vi "Find Gamma.vi"(8 "error in (no error)":errorcluster, 10 "IK Parameters":T2, 11 "Data in":T1={"link 1 angle"=0.0, "link 2 angle"=0.0, "link 1 length"=0.0, "link 2 length"=0.0, "Current arm location"=[{"X"=0.0, "Y"=0.0}, {"X"=-37.249783598972314, "Y"=33.353464914904016}, {"X"=-74.49956719794463, "Y"=66.70692982980803}], "Link Picture"=bytes[1162], "Desired Location"={"Desired X"=0.0, "Desired Y"=0.0}, "Next Location"={"Next X"=0.0, "Next Y"=0.0}, "Error"={"Joint1 error"=0.0, "Joint2 error"=0.0}, "tdms data"=refnum, "de/dt"={"joint1 de/dt"=0.0, "joint2 de/dt"=0.0}, "Voltages"={"Joint1 voltage"=0.0, "Joint2 voltage"=0.0}, "Time"=0.0, "dt"=0.0, "counts/rev"=0.0, "kp"=0.0, "kd"=0.0, "ki"=0.0, "Int(error)"={"joint1 int(e)"=0.0, "joint2 int(e)"=0.0}, "Desired angles"={"theta 1"=0.0, "theta 2"=0.0}, "Current counts"={"theta 1"=0.0, "theta 2"=0.0}, "Desired Counts"={"theta 1"=0.0, "theta 2"=0.0}, "Preivous Error"={"Joint1 Previous error"=0.0, "Joint2 Previous error"=0.0}, "Counts/s"=0.0, "Correct counter"=0}) -> (0 "error out":errorcluster, 2 "IK Parameters Out":T2, 3 "Data Out":T1={"link 1 angle"=0.0, "link 2 angle"=0.0, "link 1 length"=0.0, "link 2 length"=0.0, "Current arm location"=[{"X"=0.0, "Y"=0.0}, {"X"=-37.249783598972314, "Y"=33.353464914904016}, {"X"=-74.49956719794463, "Y"=66.70692982980803}], "Link Picture"=bytes[1162], "Desired Location"={"Desired X"=0.0, "Desired Y"=0.0}, "Next Location"={"Next X"=0.0, "Next Y"=0.0}, "Error"={"Joint1 error"=0.0, "Joint2 error"=0.0}, "tdms data"=refnum, "de/dt"={"joint1 de/dt"=0.0, "joint2 de/dt"=0.0}, "Voltages"={"Joint1 voltage"=0.0, "Joint2 voltage"=0.0}, "Time"=0.0, "dt"=0.0, "counts/rev"=0.0, "kp"=0.0, "kd"=0.0, "ki"=0.0, "Int(error)"={"joint1 int(e)"=0.0, "joint2 int(e)"=0.0}, "Desired angles"={"theta 1"=0.0, "theta 2"=0.0}, "Current counts"={"theta 1"=0.0, "theta 2"=0.0}, "Desired Counts"={"theta 1"=0.0, "theta 2"=0.0}, "Preivous Error"={"Joint1 Previous error"=0.0, "Joint2 Previous error"=0.0}, "Counts/s"=0.0, "Correct counter"=0})   [LabVIEW 2016]
uses:
  Type Defs/IK parameters.ctl
  Type Defs/Host Data.ctl
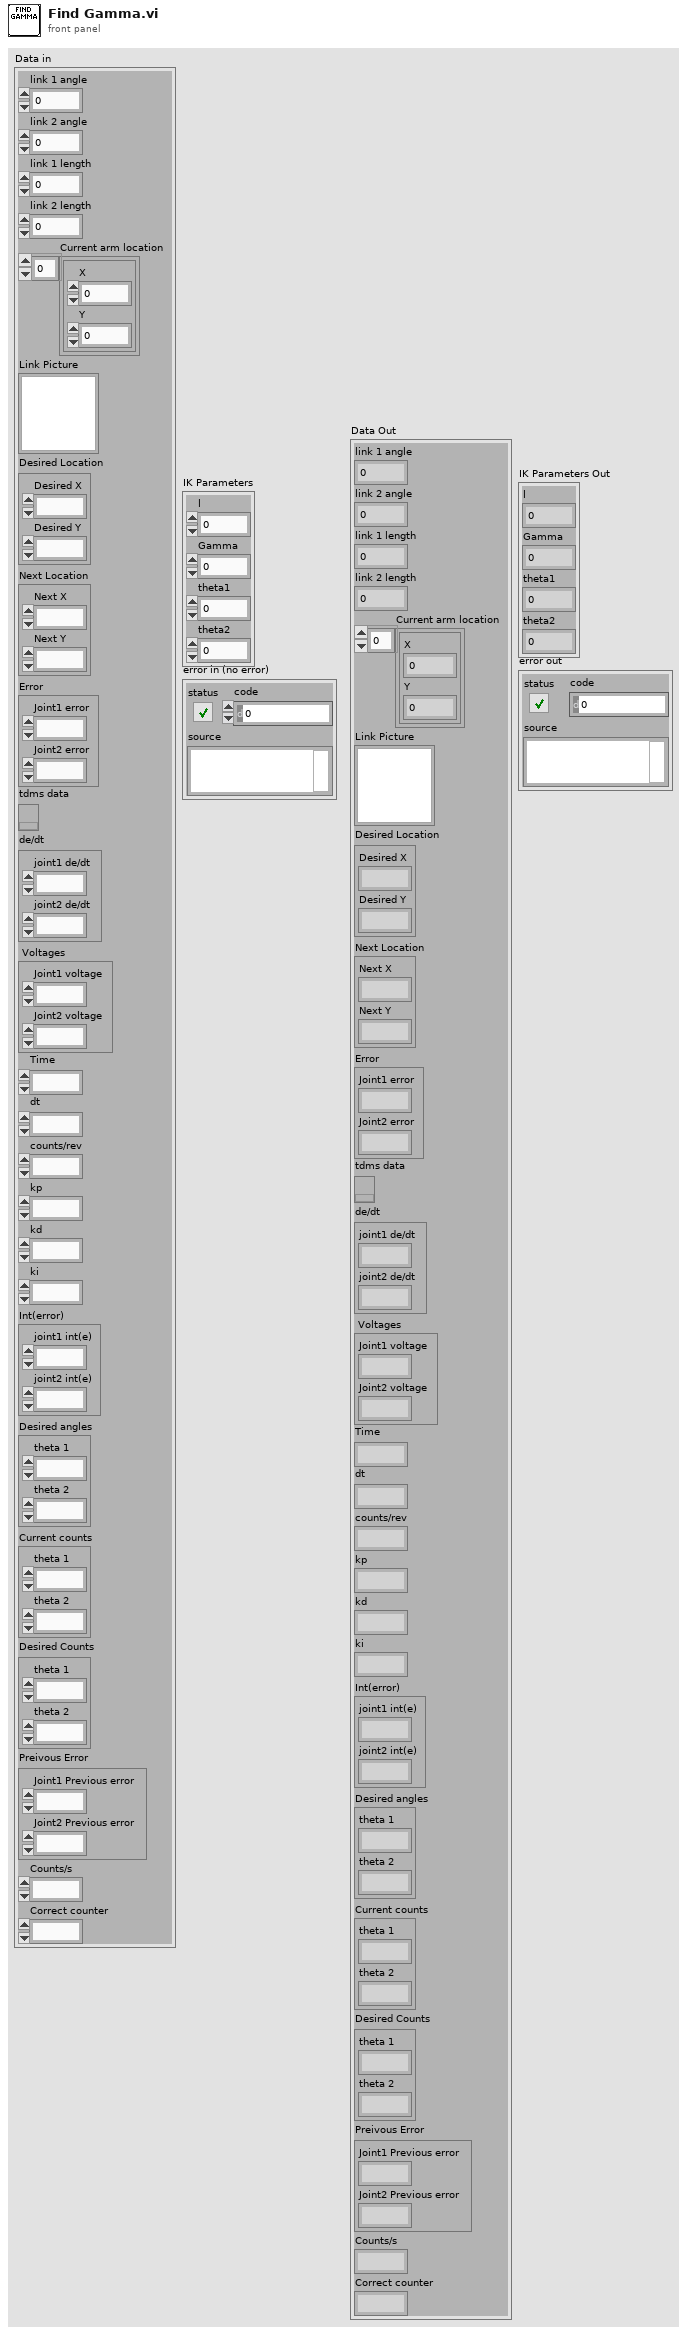
[diagram p1: front panel]
types:
  T1 = typedef "Host Data.ctl" = cluster{"link 1 angle":dbl, "link 2 angle":dbl, "link 1 length":dbl, "link 2 length":dbl, "Current arm location":cluster{"X":dbl, "Y":dbl}[], "Link Picture":picture, "Desired Location":cluster{"Desired X":dbl, "Desired Y":dbl}, "Next Location":cluster{"Next X":dbl, "Next Y":dbl}, "Error":cluster{"Joint1 error":dbl, "Joint2 error":dbl}, "tdms data":refnum<k34>, "de/dt":cluster{"joint1 de/dt":dbl, "joint2 de/dt":dbl}, "Voltages":cluster{"Joint1 voltage":dbl, "Joint2 voltage":dbl}, "Time":dbl, "dt":dbl, "counts/rev":dbl, "kp":dbl, "kd":dbl, "ki":dbl, "Int(error)":cluster{"joint1 int(e)":dbl, "joint2 int(e)":dbl}, "Desired angles":cluster{"theta 1":dbl, "theta 2":dbl}, "Current counts":cluster{"theta 1":dbl, "theta 2":dbl}, "Desired Counts":cluster{"theta 1":dbl, "theta 2":dbl}, "Preivous Error":cluster{"Joint1 Previous error":dbl, "Joint2 Previous error":dbl}, "Counts/s":dbl, "Correct counter":i32}
  T2 = typedef "IK parameters.ctl" = cluster{"l":dbl, "Gamma":dbl, "theta1":dbl, "theta2":dbl}
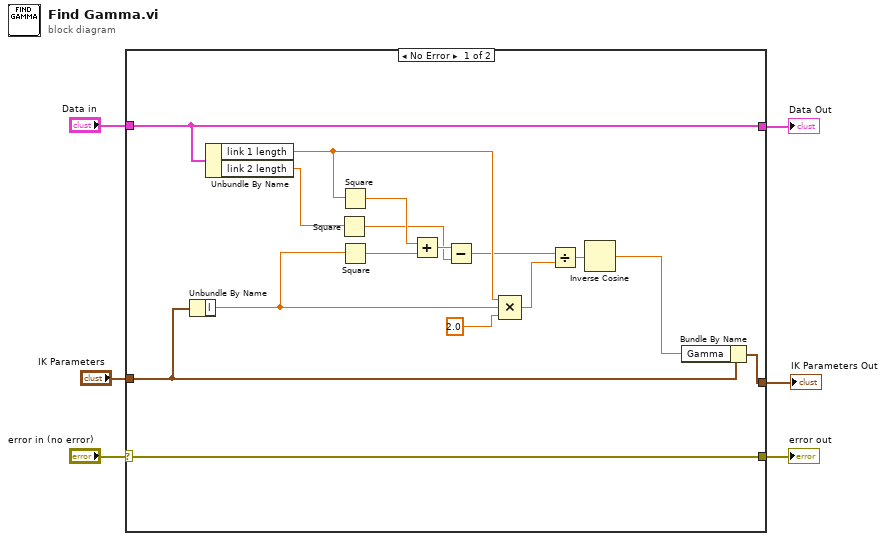
[diagram p0: block diagram]
diagram:
  n1 = case shown="No Error" "error in (no error)" {
    selector: "error in (no error)" -> [w21 w25]
    tunnel: [w21 w25] -> w5
    tunnel: "Data in" -> [w22 w24]
    tunnel: "IK Parameters" -> [w8 w23]
    tunnel: [w22 w24] -> w2
    tunnel: [w7 w23] -> w1
    frame No Error {
      n2 = Unbundle By Name(w8) -> ("l"=w14:dbl)
      n3 = Unbundle By Name(w22) -> ("link 1 length"=w15:dbl, "link 2 length"=w20:dbl)
      n4 = Square(x=w20) -> (x^2=w16:dbl)
      n5 = Square(x=w15) -> (x^2=w19:dbl)
      n6 = Square(x=w14) -> (x^2=w18:dbl)
      n7 = Add(x=w19, y=w18) -> (x+y=w17:dbl)
      n8 = Subtract(x=w17, y=w16) -> (x-y=w12:dbl)
      n9 = Compound Arithmetic op=MULTIPLY(w15, w14, 2.0) -> (w11:dbl)
      n10 = Divide(x=w12, y=w11) -> (x/y=w10:dbl)
      n11 = Inverse Cosine(1:w10) -> (0:w9:dbl)
      n12 = Bundle By Name(cluster=w8, "Gamma"=w9) -> (w7:T2)
    }
    frame Error {
    }
  }
  "error out" <- w5
  "IK Parameters Out" <- w1
  "Data Out" <- w2
